vi "Delay.vi"(8 "error in (no error)":errorcluster, 10 "Delay Time (0 ms)":u32 max=100000, 11 "VISA resource name":refnum<visa-resource-name>) -> (0 "error out":errorcluster, 3 "VISA resource name out":refnum<visa-resource-name>)   [LabVIEW 2020, in "BK Precision 911X Series.lvlib"]
uses:
  BK Precision 911X Series.lvlib
panel:
  # "ms"
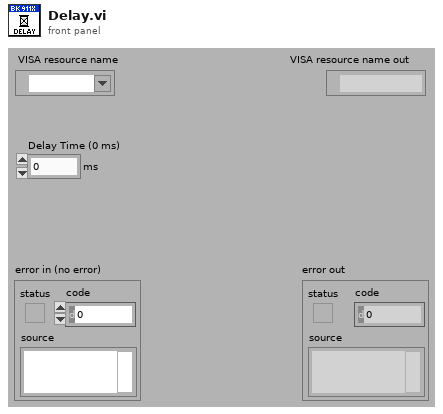
[diagram p1: front panel]
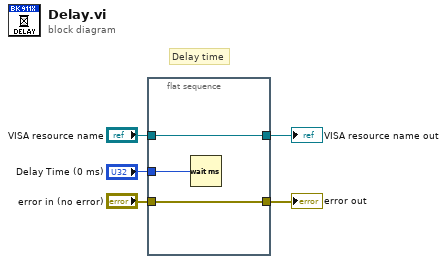
[diagram p0: block diagram]
diagram:
  # "Delay time"
  n1 = flat-sequence {
    tunnel: "Delay Time (0 ms)" -> [w8]
    tunnel: [w7] -> w4
    tunnel: "VISA resource name" -> [w7]
    tunnel: [w6] -> w2
    tunnel: "error in (no error)" -> [w6]
    frame #0 {
      n2 = Wait (ms)(milliseconds to wait=w8) -> ()  [unwired: 1 out]
    }
  }
  "VISA resource name out" <- w4
  "error out" <- w2
